vi "Subsystem Sequencer Controller.vi"(8 "error in":errorcluster) -> ()   [LabVIEW 2018]
doc: "This VI executes continuously carrying out the current operation and responding to updates or new operations. It will often contain the timing or control code that is difficult to place directly in TeleOp. This VI generally opens all sensors and motors and isolates the rest of the robot code from knowing how the operations are carried out."
uses:
  <vilib>/Rock Robotics/WPI/Framework/Completion Status.ctl
  Subsystem Sequencer Setpoints.ctl
  Subsystem Sequencer Operations.ctl
  All Commands.ctl
panel:
  in  "In Position":dbl=105.0 format="%#_13g"
  in  "Pickup Position":dbl format="%#_13g"
  out "Value":dbl
  out "Cmd":T1
  in  "Interactive Values":T2
  out "Current\nCmd":string
  in  "Buttons":cluster{"Execute Cmd":bool, "Abort Cmd":bool}
  out "Command Timing":cluster{"Start Time (ms)":u32, "Iterations":i32}
  out "Status":T4
  # "Interactive Command: You may fill in the settings for a command\nand schedule it with the Execute button. You can observe and abort\nany command while fine tuning the code for the controller."
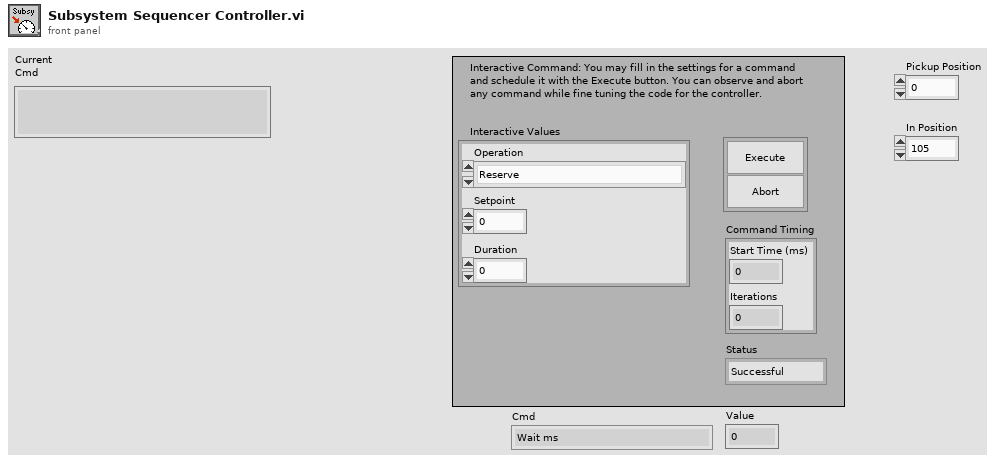
[diagram p1: front panel]
types:
  T1 = typedef "All Commands.ctl" = enum16{"Wait ms", "Drive - Stop Driving", "Drive - Drive Distance Straight", "Elevator - Elevator Stop", "Elevator - Elevator Set Position Wait", "Elevator - Elevator Set Position Start", "Elevator - Wait for Down Fast", "Wrist - Up", "Wrist - Down", "Wrist - Set Position", "Beak - Extend", "Beak - Retract", "Beak - Open", "Beak - Close", "Roller - Off", "Roller - Out", "Roller - In"}
  T2 = typedef "Subsystem Sequencer Setpoints.ctl" = cluster{"Operation":T3, "Setpoint":dbl, "Duration":dbl}
  T3 = typedef "Subsystem Sequencer Operations.ctl" = enum16{"Reserve", "Read Current", "Run Sequence"}
  T4 = typedef "Completion Status.ctl" = enum16{"Successful", "Aborted", "Incomplete"}
  T5 = typedef "Command Status Info.ctl" = cluster{"Name":string, "Status":T4, "notifier out":T6}
  T6 = typedef "Completion Notifier.ctl" = refnum<notifier>
  T7 = cluster{"Current Command":T2, "Command Timing":cluster{"Start Time (ms)":u32, "Iterations":i32}, "Command Arguments":cluster{"Command Info":T5, "Description":string, "Default Command":T2, "queue out":refnum<queue>, "Subsystem Name":string}}
  T8 = typedef "Sequencer Type.ctl" = cluster{"Cmd":T1, "Value":dbl}
  T9 = typedef "Elevator Telemetry.ctl" = cluster{"Is Moving?":bool, "Setpoint":dbl, "Velocity":dbl, "Position":dbl, "Top Limit":bool, "Bottom Limit":bool, "Applied Output":dbl}
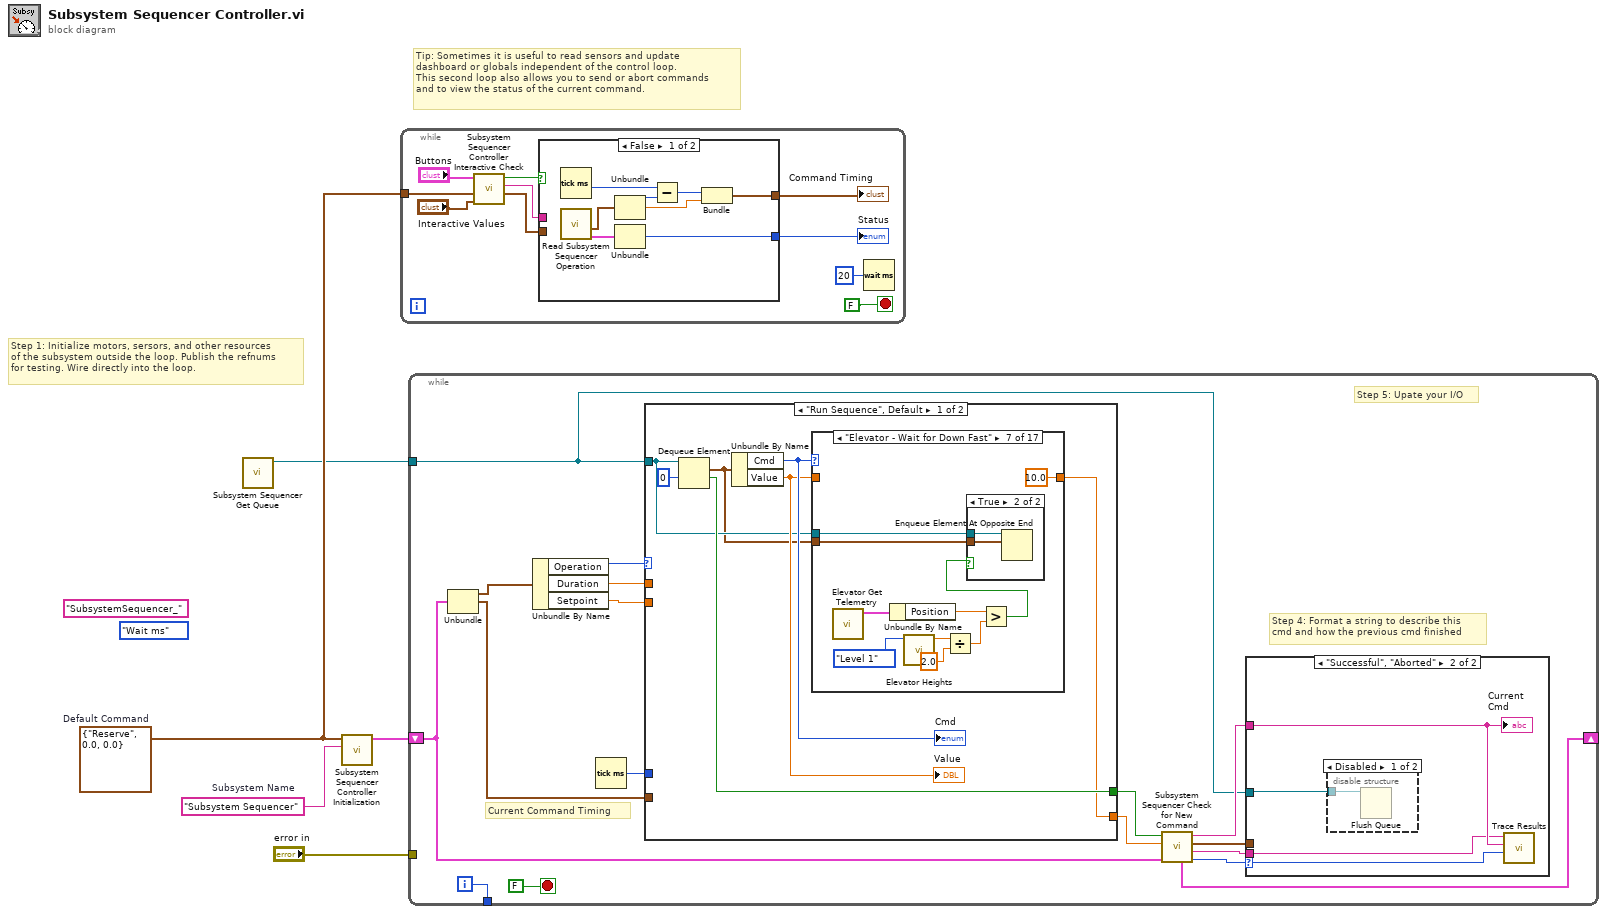
[diagram p0: block diagram]
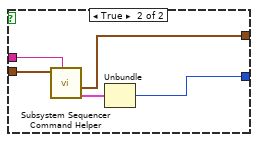
[diagram p2: hidden frame]
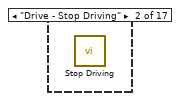
[diagram p6: hidden frame]
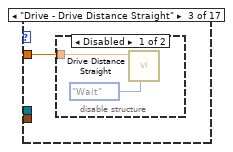
[diagram p7: hidden frame]
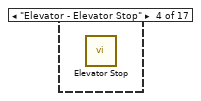
[diagram p9: hidden frame]
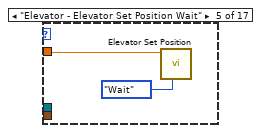
[diagram p10: hidden frame]
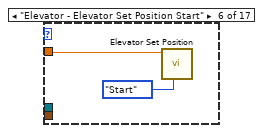
[diagram p11: hidden frame]
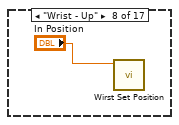
[diagram p13: hidden frame]
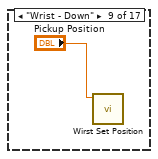
[diagram p14: hidden frame]
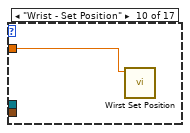
[diagram p15: hidden frame]
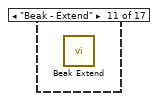
[diagram p16: hidden frame]
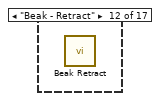
[diagram p17: hidden frame]
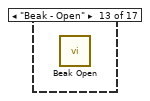
[diagram p18: hidden frame]
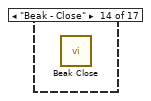
[diagram p19: hidden frame]
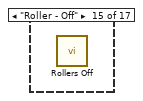
[diagram p20: hidden frame]
diagram:
  (unwired) "SubsystemSequencer_" ("name (unnamed)")
  (unwired) All_Commands."Wait ms" ("Cmd")
  w2 = T2 {"Operation"=enum."Reserve", "Setpoint"=0.0, "Duration"=0.0}  # Default Command
  w3 = "Subsystem Sequencer"  # Subsystem Name
  # "Tip: Sometimes it is useful to read sensors and update\ndashboard or globals independent of the control loop.\nThis second loop also allows you to send or abort commands\nand to view the status of the current command."
  # "Step 1: Initialize motors, sersors, and other resources\nof the subsystem outside the loop. Publish the refnums\nfor testing. Wire directly into the loop."
  n1 = call "Subsystem Sequencer Get Queue.vi"() -> ("queue out"=w1:refnum<queue>)  [unwired: 10 in, 1 out]
  n2 = call "Subsystem Sequencer Controller Initialization.vi"("Subsystem Name"=w3, "Default Command"=w2) -> ("Current Command"=w4:T7)  [unwired: 9 in]
  n3 = while {
    tunnel: w2 -> [w12]
    stop <- FALSE stop-if-true
    n4 = call "Subsystem Sequencer Controller Interactive Check.vi"("Interactive Command in"="Interactive Values", "Default Command"=w12, "Buttons"="Buttons") -> ("Interactive Command out"=w9:T2, "Trace String"=w10:string, "Schedule"=w11:bool)  [unwired: 6 in]
    n5 = case shown="False" w11 {
      tunnel: [w23 w28] -> w8
      tunnel: w9 -> [_ w26]
      tunnel: [w19 w24] -> w7
      tunnel: w10 -> [_ w27]
      frame False {
        n6 = Tick Count (ms)() -> (millisecond timer value=w18:u32)
        n7 = call "Read Subsystem Sequencer Operation.vi"() -> ("Command Info"=w16:T5, "SubSystem Data"=w17:T2)  [unwired: 9 in, 1 out]
        n8 = Unbundle(w17) -> ("Operation"=w22:T3, "Setpoint"=w20:dbl)  [unwired: 1 out]
        n9 = Unbundle(w16) -> ("Status"=w23:T4)  [unwired: 2 out]
        n10 = Subtract(x=w18, y=w22) -> (x-y=w21:u32)
        n11 = Bundle(w21, "Setpoint"=w20) -> (w19:cluster{u32, "Setpoint":dbl})  [unwired: 1 in]
      }
      frame True {
        n12 = call "Subsystem Sequencer Command Helper.vi"("Description"=w27, "SubSystem Data"=w26) -> ("Command Info Out"=w25:T5, "Command Timing"=w24:cluster{"Start Time (ms)":u32, "Iterations":i32})  [unwired: 7 in, 1 out]
        n13 = Unbundle(w25) -> ("Status"=w28:T4)  [unwired: 2 out]
      }
    }
    "Status" <- w8
    "Command Timing" <- w7
    n14 = Wait (ms)(milliseconds to wait=u32 20) -> ()  [unwired: 1 out]
  }
  n15 = while {
    shift-right: [w37] -> _
    shift-left: w4 -> [w30]
    tunnel: [w44] -> _
    tunnel: "error in" -> [_]
    tunnel: w1 -> [w29]
    i -> [w44]
    stop <- FALSE stop-if-true
    # "Step 5: Upate your I/O"
    # "Step 4: Format a string to describe this\ncmd and how the previous cmd finished"
    # "Current Command Timing"
    n16 = Unbundle(w30) -> ("Current Command"=w43:T2, "Command Timing"=w39:cluster{"Start Time (ms)":u32, "Iterations":i32})  [unwired: 1 out]
    n17 = Unbundle By Name(w43) -> ("Operation"=w42:T3, "Duration"=w41:dbl, "Setpoint"=w38:dbl)
    n18 = Tick Count (ms)() -> (millisecond timer value=w40:u32)
    n19 = case shown="\"Run Sequence\", Default" w42 {
      tunnel: [w53 w82] -> w35
      tunnel: [w56 FALSE ("ignore previous (F)")] -> w36
      tunnel: w39 -> [_ _]
      tunnel: w41 -> [_ _]
      tunnel: w40 -> [_ _]
      tunnel: w38 -> [_ _]
      tunnel: w29 -> [w52 _]
      frame "Run Sequence", Default {
        n20 = Dequeue Element(queue=w52, timeout in ms (-1)=0) -> (element=w51:T8, timed out?=w56:bool)  [unwired: 1 in, 2 out]
        n21 = Unbundle By Name(w51) -> ("Cmd"=w55:T1, "Value"=w54:dbl)
        "Cmd" <- w55
        "Value" <- w54
        n22 = case shown="\"Elevator - Wait for Down Fast\"" w55 {
          tunnel: w54 -> [w58 _ w59 _ w63 w65 _ _ _ w80 _ _ _ _ _ _ _]
          tunnel: [w58 _ _ _ _ _ 10.0 ("Value") _ _ _ _ _ _ _ _ _ _] -> w53
          tunnel: w52 -> [_ _ _ _ _ _ w75 _ _ _ _ _ _ _ _ _ _]
          tunnel: w51 -> [_ _ _ _ _ _ w74 _ _ _ _ _ _ _ _ _ _]
          frame "Wait ms", Default {
          }
          frame "Drive - Stop Driving" {
            n23 = call "Stop Driving.vi"() -> ()  [unwired: 11 in, 1 out]
          }
          frame "Drive - Drive Distance Straight" {
            n24 = disable-structure shown="Disabled" {
              disable-tunnel: w59 -> [w61 _]
              frame Disabled {
                n25 = call "Drive Distance Straight.vi"("Synchronication"=enum16{"Start", "Wait"}."Wait", "Distance"=w61) -> ()  [unwired: 9 in, 1 out]
              }
              frame Enabled {
              }
            }
          }
          frame "Elevator - Elevator Stop" {
            n26 = call "Elevator Stop.vi"() -> ()  [unwired: 11 in, 1 out]
          }
          frame "Elevator - Elevator Set Position Wait" {
            n27 = call "Elevator Set Position.vi"("Synchronization"=enum16{"Start", "Wait"}."Wait", "Setpoint"=w63) -> ()  [unwired: 9 in, 1 out]
          }
          frame "Elevator - Elevator Set Position Start" {
            n28 = call "Elevator Set Position.vi"("Synchronization"=enum16{"Start", "Wait"}."Start", "Setpoint"=w65) -> ()  [unwired: 9 in, 1 out]
          }
          frame "Elevator - Wait for Down Fast" {
            n29 = call "Elevator Get Telemetry.vi"() -> ("Telemetry"=w72:T9)  [unwired: 11 in]
            n30 = Unbundle By Name(w72) -> ("Position"=w71:dbl)
            n31 = call "Elevator Heights.vi"("Level"=enum16{"Level 1", "Level 2", "Level 3"}."Level 1") -> ("Height"=w70:dbl)  [unwired: 10 in]
            n32 = Divide(x=w70, y=2.0) -> (x/y=w69:dbl)
            n33 = Greater?(x=w71, y=w69) -> (0:w68:bool)
            n34 = case shown="True" w68 {
              tunnel: w75 -> [_ w77]
              tunnel: w74 -> [_ w76]
              frame False {
              }
              frame True {
                n35 = Enqueue Element At Opposite End(queue=w77, element=w76) -> ()  [unwired: 2 in, 3 out]
              }
            }
          }
          frame "Wrist - Up" {
            n36 = call "Wirst Set Position.vi"("Setpoint (Degrees)"="In Position") -> ()  [unwired: 10 in, 1 out]
          }
          frame "Wrist - Down" {
            n37 = call "Wirst Set Position.vi"("Setpoint (Degrees)"="Pickup Position") -> ()  [unwired: 10 in, 1 out]
          }
          frame "Wrist - Set Position" {
            n38 = call "Wirst Set Position.vi"("Setpoint (Degrees)"=w80) -> ()  [unwired: 10 in, 1 out]
          }
          frame "Beak - Extend" {
            n39 = call "Beak Extend.vi"() -> ()  [unwired: 11 in, 1 out]
          }
          frame "Beak - Retract" {
            n40 = call "Beak Retract.vi"() -> ()  [unwired: 11 in, 1 out]
          }
          frame "Beak - Open" {
            n41 = call "Beak Open.vi"() -> ()  [unwired: 11 in, 1 out]
          }
          frame "Beak - Close" {
            n42 = call "Beak Close.vi"() -> ()  [unwired: 11 in, 1 out]
          }
          frame "Roller - Off" {
            n43 = call "Rollers Off.vi"() -> ()  [unwired: 11 in, 1 out]
          }
          frame "Roller - Out" {
            n44 = call "Rollers Out.vi"() -> ()  [unwired: 11 in, 1 out]
          }
          frame "Roller - In" {
            n45 = call "Rollers In.vi"() -> ()  [unwired: 11 in, 1 out]
          }
        }
      }
      frame "Reserve" {
        w82 = 100.0  # Infinite
        # "For debugging the sensor"
      }
    }
    n46 = call "Subsystem Sequencer Check for New Command.vi"("Current Command"=w30, "Wait time (ms)"=w35, "Finished?"=w36) -> ("Completion"=w31:T4, "Subsystem Name"=w32:string, "Current Command"=w33:T2, "Initial Trace String"=w34:string, "NextCommand"=w37:T7)  [unwired: 4 in]
    n47 = case shown="\"Successful\", \"Aborted\"" w31 {
      selector: w31 -> [_ w49]
      tunnel: w34 -> [_ w48]
      tunnel: w33 -> [_ _]
      tunnel: w32 -> [_ w47]
      tunnel: w29 -> [_ w46]
      frame "Incomplete", Default {
        # "Continuing current command"
      }
      frame "Successful", "Aborted" {
        # "Report and setup for next command"
        n48 = disable-structure shown="Disabled" {
          disable-tunnel: w46 -> [w50 _]
          frame Disabled {
            n49 = Flush Queue(queue=w50) -> ()  [unwired: 1 in, 3 out]
          }
          frame Enabled {
          }
        }
        n50 = call <vilib>:"Trace Results.vi"("Status of previous command"=w49, "Description"=w48, "Subsystem"=w47) -> ()  [unwired: 9 in]
        "Current\nCmd" <- w48
      }
    }
  }
